vi "Read Fsetpoint (Channel F).vi"(8 "error in":errorcluster, 11 "MB_TCP session in":refnum<class "MB_Master_TCP.lvclass">) -> (0 "error out":errorcluster, 2 "Value":sgl, 3 "MB session out":refnum<class "MB_Master_TCP.lvclass">)   [LabVIEW 2024, in "Bronkhorst Flexi-Flow ModbusTCP API.lvlib"]
uses:
  Bronkhorst Flexi-Flow ModbusTCP API.lvlib
  <vilib>/Plasmionique/MB Master/MB_Master_TCP/MB_Master_TCP.lvclass
  PDU Address Float 32-bit Params--ring.ctl
  Read Float Register.vi
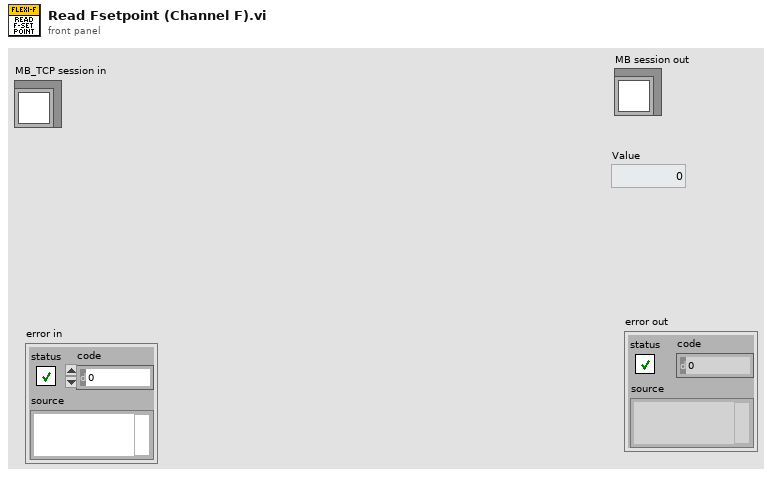
[diagram p1: front panel]
types:
  T1 = typedef "Bronkhorst Flexi-Flow ModbusTCP API.lvlib/PDU Address Float 32-bit Params--ring.ctl" = u16
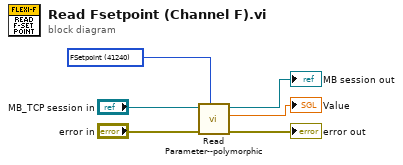
[diagram p0: block diagram]
diagram:
  w6 = T1 41240 items=["FSetpoint"=41240, "Fmeasure"=41216, "Capacity 0%"=41392, "Counter limit (Float)"=59416, "PID-Kp"=62120, "PID-Ti"=62128, "PID-Td"=62136, "Dynamic display factor"=62728, "Static display factor"=62736, "Exponential smoothing"=62752] ("PDU Address 32-bit Float")
  n1 = call-poly "Read Parameter--polymorphic.vi"("PDU Address 32-bit Float"=w6, "error in"="error in", "MB_TCP session in"="MB_TCP session in") -> ("error out"=→"error out":errorcluster, "Value"=→"Value":sgl, "MB session out"=→"MB session out":refnum<class "MB_Master_TCP.lvclass">)  [unwired: 6 in]
